vi "ZMC Make Zar2.vi"(6 "uid":u32, 7 "pPass":string, 8 "error in (no error)":errorcluster caption="错误输入（无错误）", 9 "pZarfilename":string, 10 "pBasDir":string, 11 "pzpj":u32) -> (0 "error out":errorcluster caption="错误输出", 2 "function return":i32, 3 "pzpj out":u32)   [LabVIEW 2015, in "zauxdll.lvlib"]
doc: "int32 __stdcall ZMC_MakeZar2(void *pzpj,const char *pBasDir, const char* pZarfilename, const char *pPass, uint32 uid);"
uses:
  zauxdll.lvlib
  zmotion.dll
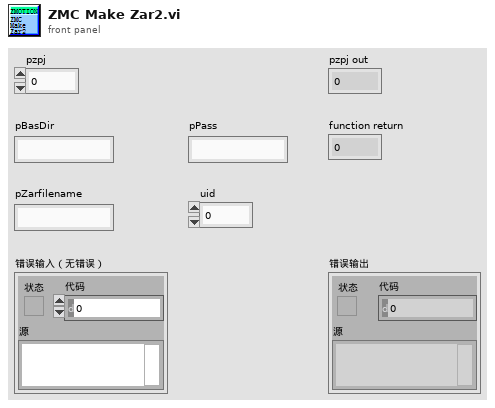
[diagram p1: front panel]
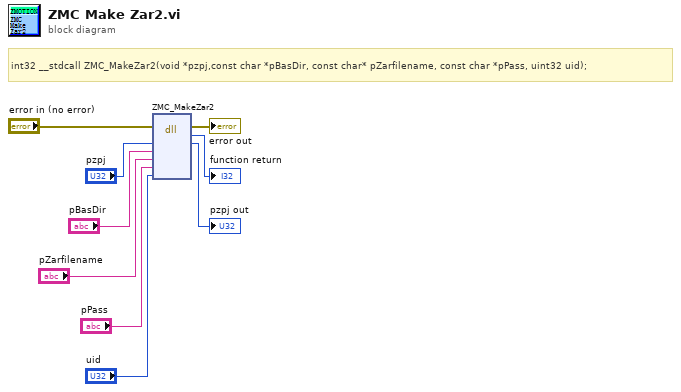
[diagram p0: block diagram]
diagram:
  # "int32 __stdcall ZMC_MakeZar2(void *pzpj,const char *pBasDir, const char* pZarfilename, const char *pPass, uint32 uid);"
  n1 = dll-call lib="C:/Users/VIC/Desktop/GOGORO_SA/system/LLB/zmotion/zaux/zmotion.*" fn="ZMC_MakeZar2"(error in="error in (no error)", "pzpj"="pzpj", "pBasDir"="pBasDir", "pZarfilename"="pZarfilename", "pPass"="pPass", "uid"="uid") -> (error out=→"error out":errorcluster, →"function return":i32, "pzpj"=→"pzpj out":u32)  [unwired: 6 in, 1 out]
